vi "8_Calculate Y_solution.vi"(11 "x":dbl) -> (3 "y":dbl)   [LabVIEW 2014]
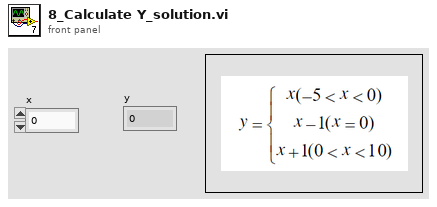
[diagram p1: front panel]
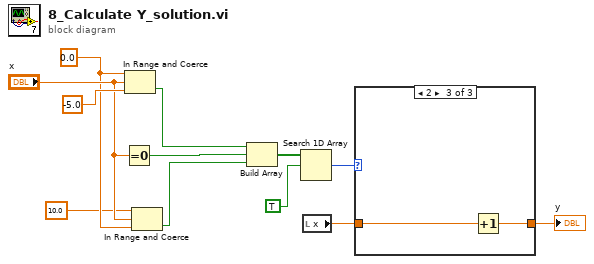
[diagram p0: block diagram]
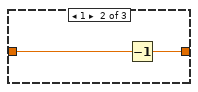
[diagram p3: hidden frame]
diagram:
  w10 = 0.0
  n1 = Equal To 0?(x="x") -> (x = 0?=w7:bool)
  n2 = In Range and Coerce(upper limit=w10, x="x", lower limit=-5.0) -> (In Range?=w8:bool)  [unwired: 1 out]
  n3 = In Range and Coerce(upper limit=10.0, x="x", lower limit=w10) -> (In Range?=w6:bool)  [unwired: 1 out]
  n4 = Build Array(w8, w7, w6) -> (w5:bool[])
  n5 = Search 1D Array(1D array=w5, element=TRUE) -> (index of element=w3:i32)  [unwired: 1 in]
  n6 = local read "x"() -> (w1:dbl)
  n7 = case shown="2" w3 {
    tunnel: [w13 w15 w17] -> w2
    tunnel: w1 -> [w13 w14 w16]
    frame 0, Default {
    }
    frame 1 {
      n8 = Decrement(x=w14) -> (x-1=w15:dbl)
    }
    frame 2 {
      n9 = Increment(x=w16) -> (x+1=w17:dbl)
    }
  }
  "y" <- w2
